vi "Output Wrist.vi"(11 "TeleOp Data Cluster":T1={"Drive Forward Input "=0.0, "Drive Twist Input"=0.0, "Drive Output"=0.0, "Drivetwist Output"=0.0, "Left Joystick Buttons"=[], "Left Joystick Axis"=[], "Right Joystick Axis"=[0.0, -0.007874015748031496, 0.0, -1.0], "Right Joystick Button"=[FALSE, FALSE, FALSE, FALSE, FALSE, FALSE, FALSE, FALSE, FALSE, FALSE, FALSE, FALSE], "Arm Encoder"=-20.0, "Left Drive Encoder"=0.0, "Right Drive Encoder"=36963.0, "Gyro Angle "=16.259765625, "Arm Joystick Output  "=-0.003937007874015748, "Line Follower L, C, R "=[TRUE, TRUE, TRUE], "Line follow?"=FALSE, " Climb Solenoid"=FALSE, "Wrist Encoder Count"=0.0, "Wrist Joystick Output"=0.0, "Ball Encoder Count"=0.0, "Ball Output"=0.0, "Climb Encoder"=0.0, "Climb Motor Output"=0.0, " Hatch Solenoid"=FALSE, "Arm Setpoint "=6.0, "Wrist Setpoint "=0.0, "Arm Joystick Enabled?"=FALSE, "Wrist Joystick Enabled"=FALSE, "Vision String"="0, 0, 0, 0, 0, 0", "Left Joystick POVs"=[]}) -> ()   [LabVIEW 2018]
uses:
  TypeDefs/Teleop Data Cluster.ctl
  TypeDefs/typedef_enum_Refnums.ctl
  TypeDefs/Joystick Buttons.ctl
  <vilib>/Rock Robotics/WPI/ThirdParty/Phoenix-LabVIEW/Motor Controller/Controls/CTRE_Phoenix_MotorControl_ControlMode.ctl
  <vilib>/Rock Robotics/WPI/ThirdParty/Phoenix-LabVIEW/Motor Controller/Get/CTRE_Phoenix_MotorController_GetLimitSwitchStates.vi
  <vilib>/Rock Robotics/Network Tables/NT Write Number.vi
  <vilib>/Rock Robotics/WPI/ThirdParty/Phoenix-LabVIEW/Motor Controller/Get/CTRE_Phoenix_MotorController_GetVoltage.vi
  <vilib>/Rock Robotics/WPI/ThirdParty/Phoenix-LabVIEW/Motor Controller/Get/CTRE_Phoenix_MotorController_GetClosedLoopData.vi
  <vilib>/Rock Robotics/WPI/ThirdParty/Phoenix-LabVIEW/Motor Controller/Get/CTRE_Phoenix_MotorController_GetSelectedSensorData.vi
  <vilib>/Rock Robotics/Network Tables/NT Write Boolean.vi
  <vilib>/ptbypt/NI_PtbyPt.lvlib
panel:
  in  "test setpt":i32
  in  "Setpoint 0":i32=-75
  in  "Top: Button; Bot: test":bool=TRUE
  in  "Setpoint 2":i32=600
  in  "Setpoint 1":i32=100
  out "Angle Out":dbl=22.5
  out "velocity Chart":i32(graph)
  out "Encoder Count":dbl
  out "Quadrature Velocity":i32
  in  "joystick scale factor":dbl=0.3
  in  "joystick upper limit":dbl=0.3 format="%#_13g"
  in  "joystick lower limit":dbl=-0.3 format="%#_13g"
  in  "P":dbl
  in  "I":dbl
  in  "D":dbl
  in  "slotIdx":i32
  out "Encoder Graph":dbl[][](graph)=[[-75.0, 0.0]]
  out "Closed-loop Error":i32=-75
  out "Error Derivative":dbl
  out "Integral Accumulator":dbl=-4611840.0
  out "Closed-loop Target":dbl=-0.075
  out "Percent Output":dbl
  in  "Cruise Angular Velocity raw":dbl=200.0 format="%#_13g"
  in  "Maximum Angular Accel raw":dbl=500.0 format="%#_13g"
  out "Closed Loop Target (deg)":dbl=-50.00164794921875
  out "Closed Loop Error (deg)":dbl=-51.64794921875
  in  "F":dbl
  in  "Arbitrary Feed Forward at 0":dbl
  in  "dt":u32
  in  "Reset Encoder":bool
  in  "joystick control? OR Thumb":bool
  # "top:  button mode"
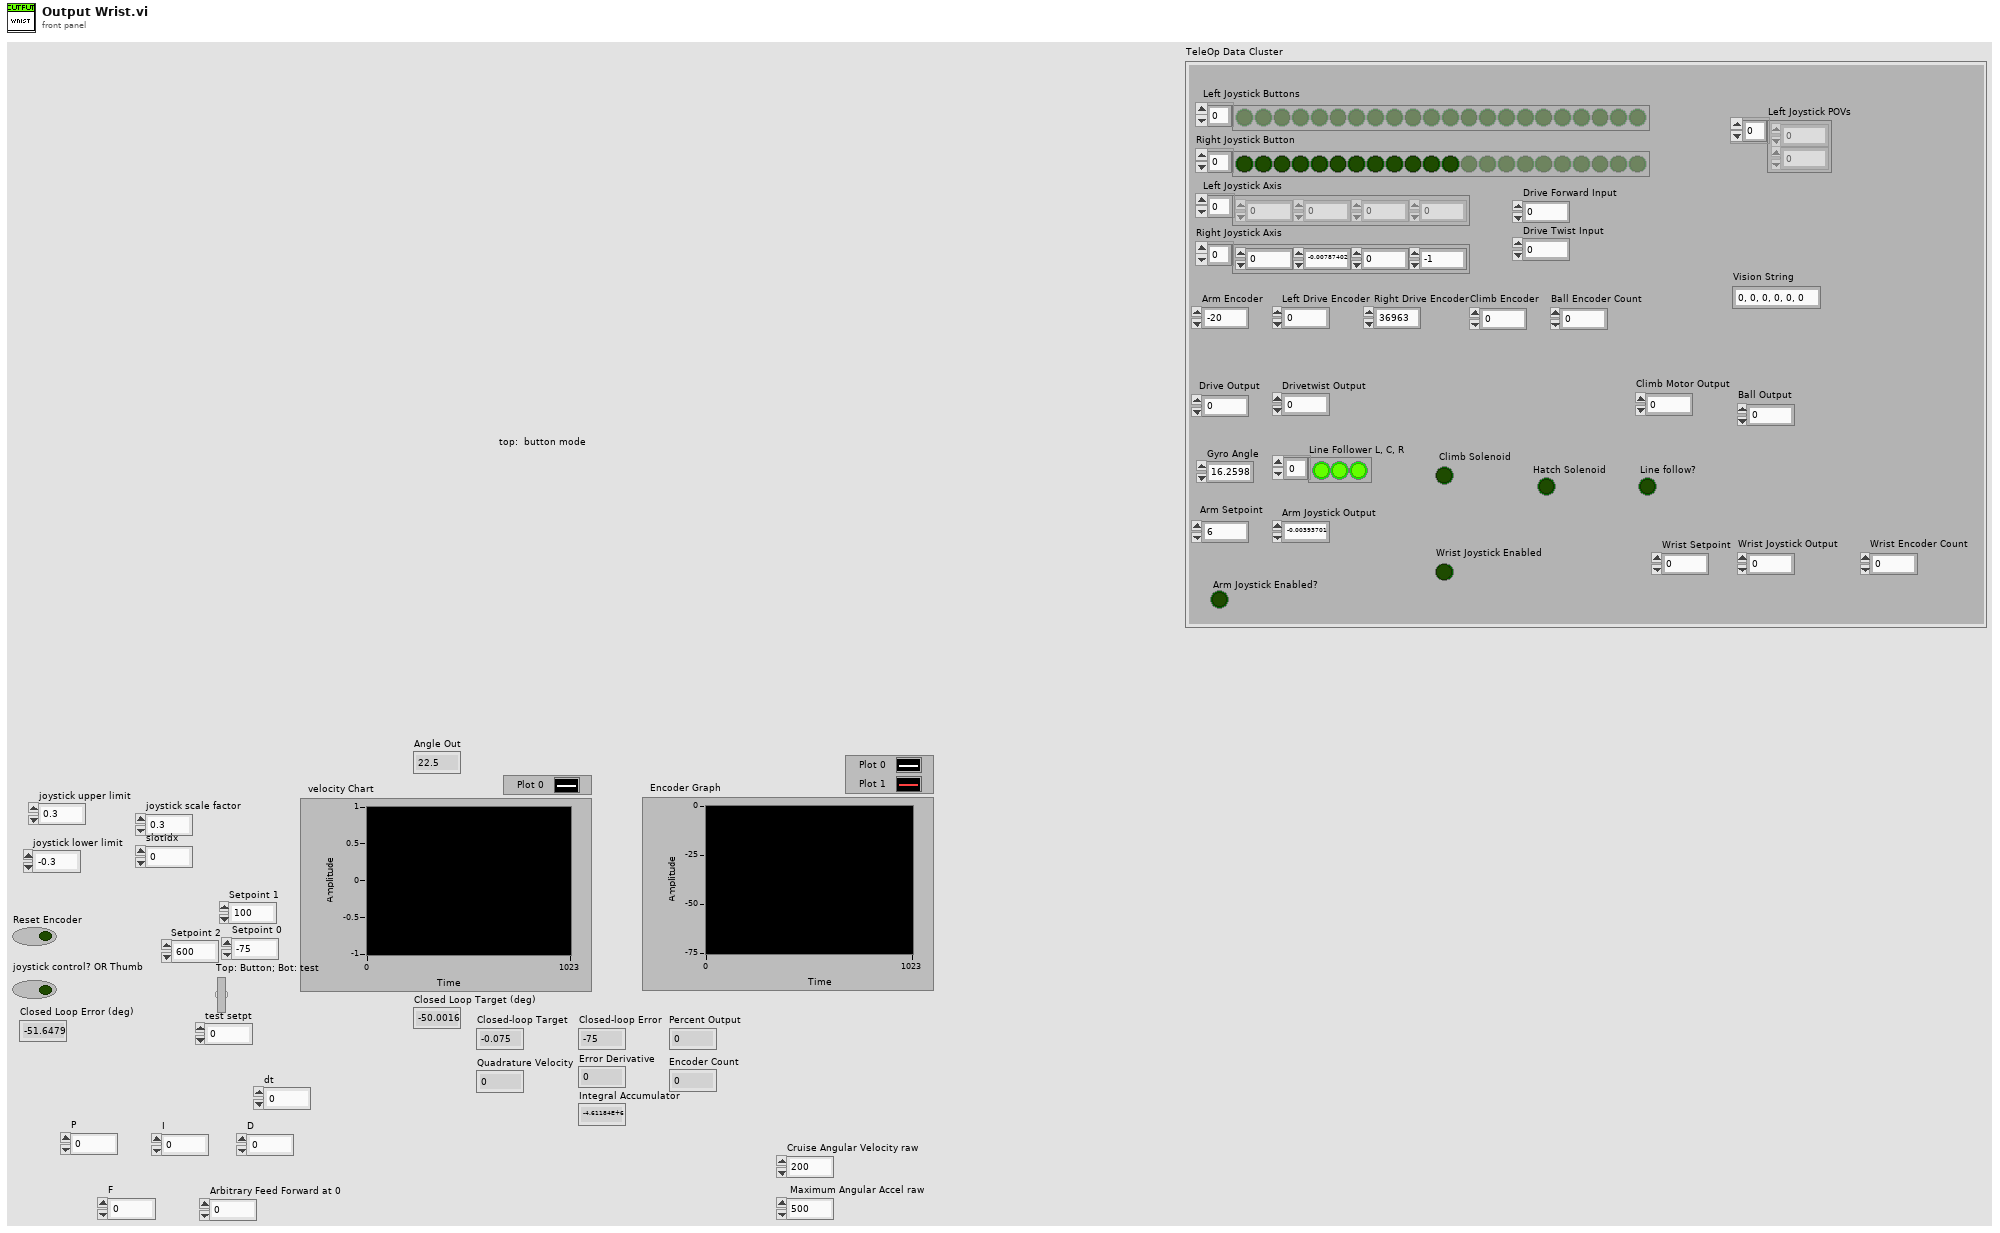
[diagram p1: front panel]
types:
  T1 = typedef "Teleop Data Cluster.ctl" = cluster{"Drive Forward Input ":dbl, "Drive Twist Input":dbl, "Drive Output":dbl, "Drivetwist Output":dbl, "Left Joystick Buttons":bool[], "Left Joystick Axis":dbl[], "Right Joystick Axis":dbl[], "Right Joystick Button":bool[], "Arm Encoder":dbl, "Left Drive Encoder":dbl, "Right Drive Encoder":dbl, "Gyro Angle ":dbl, "Arm Joystick Output  ":dbl, "Line Follower L, C, R ":bool[], "Line follow?":bool, " Climb Solenoid":bool, "Wrist Encoder Count":dbl, "Wrist Joystick Output":dbl, "Ball Encoder Count":dbl, "Ball Output":dbl, "Climb Encoder":dbl, "Climb Motor Output":dbl, " Hatch Solenoid":bool, "Arm Setpoint ":dbl, "Wrist Setpoint ":dbl, "Arm Joystick Enabled?":bool, "Wrist Joystick Enabled":bool, "Vision String":string, "Left Joystick POVs":i16[]}
  T2 = typedef "Joystick Buttons.ctl" = enum16{"Trigger", "Thumb", "Top 3", "Top 4", "Top 5", "Top 6", "Bottom 7", "Bottom 8", "Bottom 9", "Bottom 10", "Bottom 11", "Bottom 12"}
  T3 = typedef "typedef_enum_Refnums.ctl" = enum16{"Ball_Encoder", "Ball_Motor", "Camera", "Linefollow_3", "Linefollow_2", "Linefollow_1", "Gyro", "Hatch_Solenoid", "Climb_Back_Solenoid", "Arm_Encoder", "Arm_Motor", "Lift_Encoder", "Drive", "Drive_Motor_R", "Drive_Motor_L", "Drive_Encoder_R", "Drive_Encoder_L", "Joy_R", "Joy_L", "Wrist_Motor", "Wrist_Encoder", "Climb Upper Limit", "Climb Lower Limit ", "Climb_Front_Motor"}
  T4 = typedef "WPI_MotorControlDeviceRef.ctl" = cluster{"DeviceStatus":errorcluster, "Type":T5, "PWM":cluster{"PWM Channel":T6, "DeadBand":T7}, "CAN":cluster{"Device Number":u8, "SetOutput VI Ref":variant, "GetOutput VI Ref":variant, "Enable VI Ref":variant, "Disable VI Ref":variant, "Data":variant}, "Invert":bool, "DIO PWM":cluster{"PWM \"Enable\" Channel":T6, "DIOChannel":T8, "PWM Rate":dbl}}
  T5 = typedef "WPI_MotorControlType.ctl" = enum16{"PWM", "CAN", "DIO PWM"}
  T6 = typedef "FPGA_DIOPWMChannel.ctl" = enum8{"PWM 0", "PWM 1", "PWM 2", "PWM 3", "PWM 4", "PWM 5", "PWM 6", "PWM 7", "PWM 8", "PWM 9", "PWM MXP 0", "PWM MXP 1", "PWM MXP 2", "PWM MXP 3", "PWM MXP 4", "PWM MXP 5", "PWM MXP 6", "PWM MXP 7", "PWM MXP 8", "PWM MXP 9", "Invalid"}
  T7 = typedef "WPI_PWMDeadband.ctl" = cluster{"Name":string, "maxPositivePwm":i32, "minPositivePwm":i32, "centerPwm":i32, "maxNegativePwm":i32, "minNegativePwm":i32, "angularRange":u16}
  T8 = typedef "FPGA_DIOChannel.ctl" = enum8{"DIO 0", "DIO 1", "DIO 2", "DIO 3", "DIO 4", "DIO 5", "DIO 6", "DIO 7", "DIO 8", "DIO 9", "DIO MXP 0", "DIO MXP 1", "DIO MXP 2", "DIO MXP 3", "DIO MXP 4", "DIO MXP 5", "DIO MXP 6", "DIO MXP 7", "DIO MXP 8", "DIO MXP 9", "DIO MXP 10", "DIO MXP 11", "DIO MXP 12", "DIO MXP 13", "DIO MXP 14", "DIO MXP 15", "SPI Port CS1", "SPI Port CS2", "SPI Port CS3", "SPI Port MISO", "SPI Port MOSI", "Invalid"}
  T9 = enum16{"DemandType_Neutral", "DemandType_AuxPID", "DemandType_ArbitraryFeedForward"}
  T10 = typedef "CTRE_Phoenix_MotorControl_ControlMode.ctl" = u16
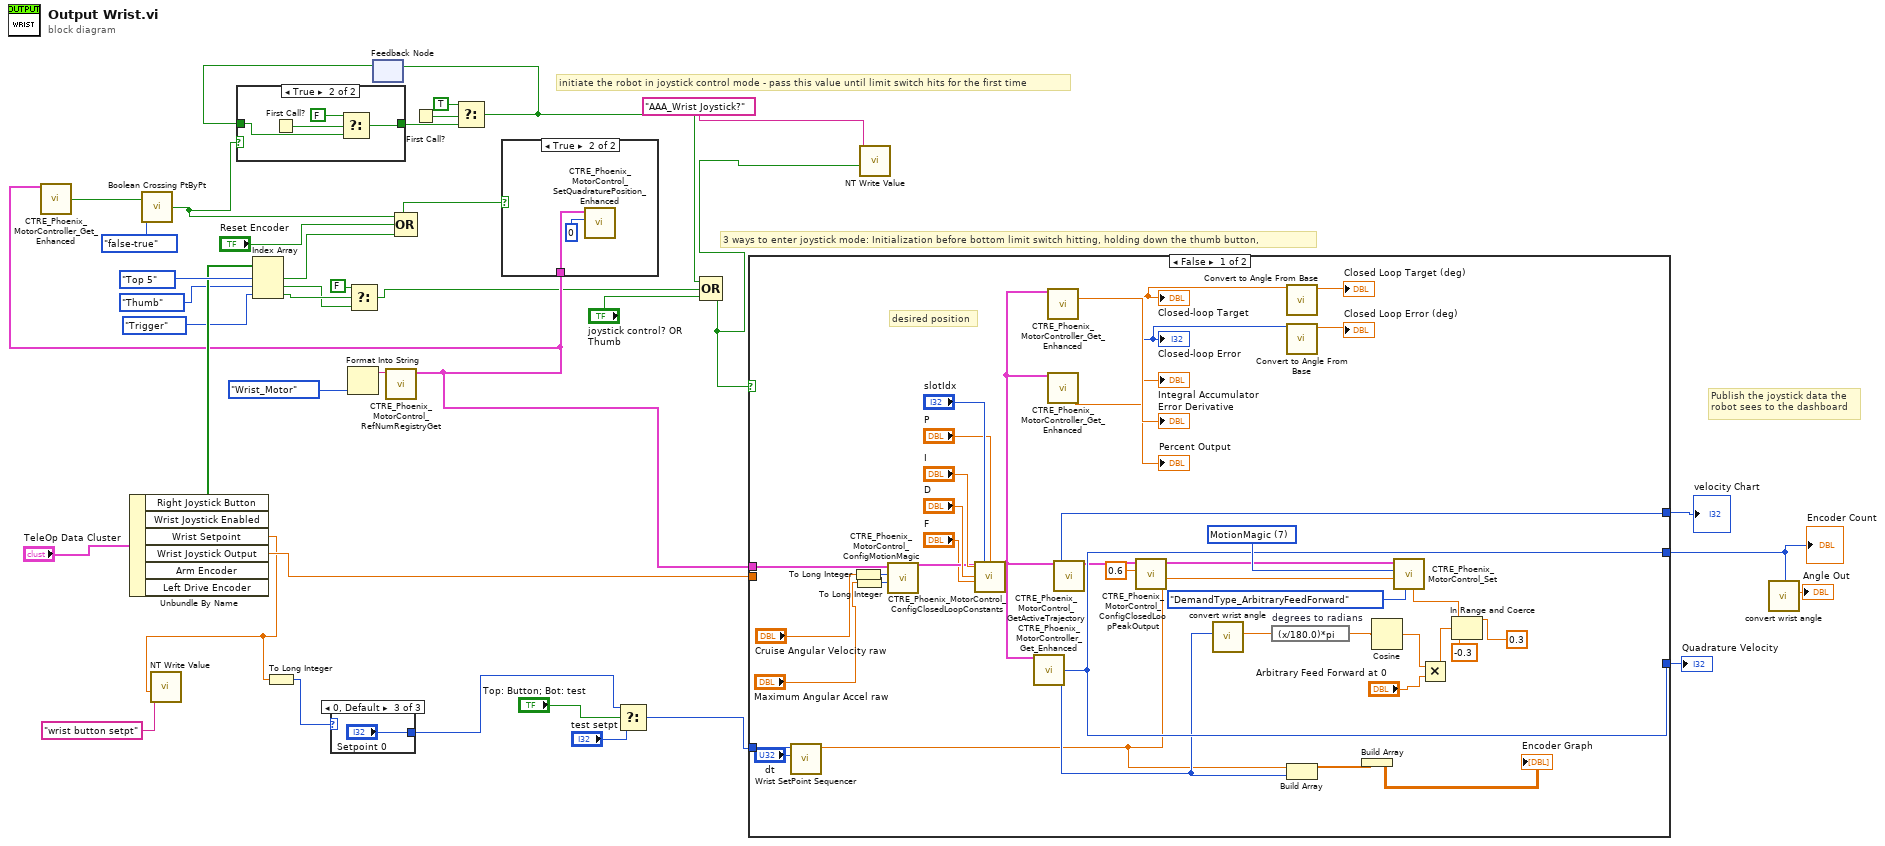
[diagram p0: block diagram]
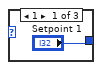
[diagram p3: hidden frame]
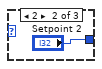
[diagram p4: hidden frame]
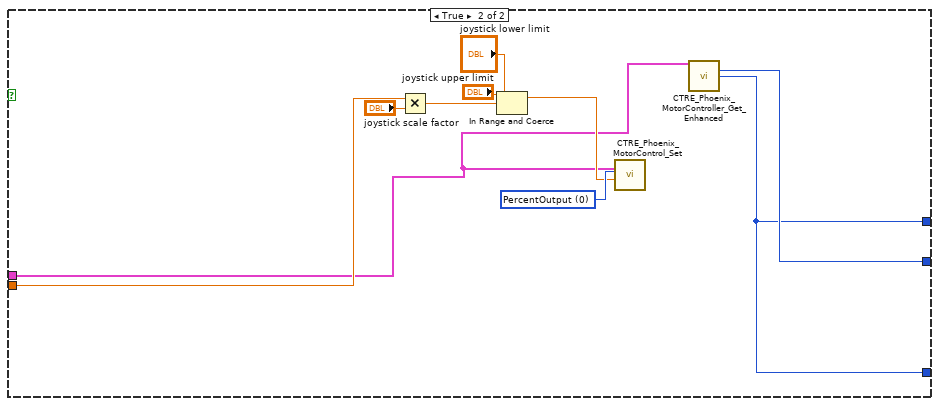
[diagram p5: hidden frame]
diagram:
  # "3 ways to enter joystick mode: Initialization before bottom limit switch hitting, holding down the thumb button,"
  # "initiate the robot in joystick control mode - pass this value until limit switch hits for the first time"
  # "Publish the joystick data the\nrobot sees to the dashboard"
  n1 = Unbundle By Name("TeleOp Data Cluster") -> ("Right Joystick Button"=w34:bool[], "Wrist Setpoint"=w24:dbl, "Wrist Joystick Output"=w28:dbl)  [unwired: 3 out]
  n2 = call-poly <vilib>:"NT Write Value.vi"("Numeric"=w24, "Name"="wrist button setpt") -> ()  [unwired: 9 in, 1 out]
  n3 = Index Array(array=w34, index #1=Joystick_Buttons."Top 5" ("Enum"), index #2=Joystick_Buttons."Thumb" ("Enum"), index #3=Joystick_Buttons."Trigger" ("Enum")) -> (element #1=w19:bool, element #2=w6:bool, element #3=w7:bool)
  n4 = To Long Integer(number=w24) -> (32bit integer=w23:i32)
  n5 = case shown="0, Default" w23 {
    tunnel: ["Setpoint 1" "Setpoint 2" "Setpoint 0"] -> w26
    frame 1 {
    }
    frame 2 {
    }
    frame 0, Default {
    }
  }
  n6 = Format Into String(typedef_enum_Refnums."Wrist_Motor" ("RefNums")) -> (resulting string=w37:string)  [unwired: 3 in, 1 out]
  n7 = Select(t=FALSE, s=w7, f=w6) -> (s? t:f=w4:bool)
  n8 = feedback #1() -> (w15:bool)  [unwired: 1 in]
  n9 = call <vilib>:"CTRE_Phoenix_MotorControl_RefNumRegistryGet.vi"("refnum name"=w37) -> ("PhoenixMotorControlDevRef"=w20:T4)  [unwired: 9 in, 1 out]
  n10 = call-poly <vilib>:"CTRE_Phoenix_MotorController_Get_Enhanced.vi"("PhoenixMotorControlDevRef"=w20) -> ("Reverse Limit Closed?"=w1:bool)  [unwired: 11 in, 3 out]
  n11 = call <vilib>:"Boolean Crossing PtByPt.vi"("direction"=enum16{"either", "false-true", "true-false"}."false-true", "input"=w1) -> ("crossing"=w17:bool)  [unwired: 1 in]
  n12 = case shown="True" w17 {
    tunnel: [w42 w43] -> w12
    tunnel: w15 -> [w42 w45]
    frame False {
    }
    frame True {
      n13 = First Call?() -> (First Call?: T/F=w46:bool)
      n14 = Select(t=FALSE, s=w46, f=w45) -> (s? t:f=w43:bool)
    }
  }
  n15 = Compound Arithmetic op=OR(w17, "Reset Encoder", w19) -> (w16:bool)
  n16 = First Call?() -> (First Call?: T/F=w14:bool)
  n17 = Select(t=TRUE, s=w14, f=w12) -> (s? t:f=w9:bool)
  n18 = feedback-in #1(w9) -> ()
  n19 = case shown="True" w16 {
    tunnel: w20 -> [_ w47]
    frame False {
    }
    frame True {
      n20 = call <vilib>:"CTRE_Phoenix_MotorControl_SetQuadraturePosition_Enhanced.vi"("New Position"=0, "PhoenixMotorControlDevRef"=w47) -> ()  [unwired: 8 in, 2 out]
    }
  }
  n21 = Select(t=w26, s="Top: Button; Bot: test", f="test setpt") -> (s? t:f=w22:i32)
  n22 = Compound Arithmetic op=OR(w9, w4, "joystick control? OR Thumb") -> (w3:bool)
  n23 = case shown="False" w3 {
    tunnel: [w76 w91] -> w32
    tunnel: [w78 w91] -> w31
    tunnel: [w76 w92] -> w30
    tunnel: w22 -> [w55 _]
    tunnel: w20 -> [w52 w89]
    tunnel: w28 -> [_ w90]
    frame False {
      w83 = T10 7 items=["PercentOutput"=0, "Position"=1, "Velocity"=2, "Current"=3, "Follower"=5, "MotionProfile"=6, "MotionMagic"=7, "MotionProfileArc"=10, "Disabled"=15] ("Control Mode")
      # "desired position"
      n24 = call "Wrist SetPoint Sequencer.vi"("dt"="dt", "SetPoint"=w55) -> ("Active SetPoint"=w54:dbl)  [unwired: 9 in]
      n25 = To Long Integer(number="Cruise Angular Velocity raw") -> (32bit integer=w74:i32)
      n26 = To Long Integer(number="Maximum Angular Accel raw") -> (32bit integer=w73:i32)
      n27 = call <vilib>:"CTRE_Phoenix_MotorControl_ConfigMotionMagic.vi"("Acceleration"=w73, "Cruise Velocity"=w74, "PhoenixMotorControlDevRef"=w52) -> ("PhoenixMotorControlDevRef"=w84:T4)  [unwired: 7 in, 1 out]
      n28 = call <vilib>:"CTRE_Phoenix_MotorControl_ConfigClosedLoopConstants.vi"("PhoenixMotorControlDevRef"=w84, "slotIdx"="slotIdx", "P"="P", "I"="I", "D"="D", "F"="F") -> ("PhoenixMotorControlDevRef"=w77:T4)  [unwired: 8 in, 1 out]
      n29 = call-poly <vilib>:"CTRE_Phoenix_MotorController_Get_Enhanced.vi"("PhoenixMotorControlDevRef"=w77) -> ("Position (Raw Sensor Units)"=w56:i32, "Velocity (Raw Sensor Units per 100 ms)"=w76:i32)  [unwired: 11 in, 2 out]
      n30 = call-poly <vilib>:"CTRE_Phoenix_MotorController_Get_Enhanced.vi"("PhoenixMotorControlDevRef"=w77) -> ("Closed-loop Target"=w71:dbl, "Closed-loop Error"=w68:i32, "Error Derivative"=→"Error Derivative":dbl, "Integral Accumulator"=→"Integral Accumulator":dbl)  [unwired: 9 in, 2 out]
      "Closed-loop Error" <- w68
      "Closed-loop Target" <- w71
      n31 = call-poly <vilib>:"CTRE_Phoenix_MotorController_Get_Enhanced.vi"("PhoenixMotorControlDevRef"=w77) -> ("Percent Output"=→"Percent Output":dbl)  [unwired: 10 in, 4 out]
      n32 = call <vilib>:"CTRE_Phoenix_MotorControl_GetActiveTrajectory.vi"("PhoenixMotorControlDevRef"=w77) -> ("PhoenixMotorControlDevRef"=w51:T4, "Velocity (Sensor Units per 100 ms)"=w78:i32)  [unwired: 10 in, 3 out]
      n33 = call <vilib>:"CTRE_Phoenix_MotorControl_ConfigClosedLoopPeakOutput.vi"("peakOutput"=0.6, "PhoenixMotorControlDevRef"=w51) -> ("PhoenixMotorControlDevRef"=w50:T4)  [unwired: 8 in, 1 out]
      n34 = call "convert wrist angle.vi"("Horizontal Encoder Ct"=w56) -> ("Angle Out"=w58:dbl)  [unwired: 9 in, 1 out]
      n35 = expression code="(x/180.0)*pi" "degrees to radians"(w58) -> (w62:dbl)
      n36 = call "Convert to Angle From Base.vi"("Horizontal Encoder Ct"=w71) -> ("Angle Out"=→"Closed Loop Target (deg)":dbl)  [unwired: 9 in, 1 out]
      n37 = call "Convert to Angle From Base.vi"("Horizontal Encoder Ct"=w68) -> ("Angle Out"=→"Closed Loop Error (deg)":dbl)  [unwired: 9 in, 1 out]
      n38 = Build Array(w54, w56) -> (w72:dbl[])
      n39 = Build Array(w72) -> (→"Encoder Graph":dbl[][])
      n40 = Cosine(x=w62) -> (cos(x)=w61:dbl)
      n41 = Multiply(x=w61, y="Arbitrary Feed Forward at 0") -> (x*y=w57:dbl)
      n42 = In Range and Coerce(upper limit=0.3, x=w57, lower limit=-0.3) -> (coerced(x)=w63:dbl)  [unwired: 1 out]
      n43 = call <vilib>:"CTRE_Phoenix_MotorControl_Set.vi"("Demand1"=w63, "DemandType"=T9."DemandType_ArbitraryFeedForward", "Output"=w54, "Control Mode"=w83, "PhoenixMotorControlDevRef"=w50) -> ()  [unwired: 5 in, 2 out]
    }
    frame True {
      w98 = T10 0 items=["PercentOutput"=0, "Position"=1, "Velocity"=2, "Current"=3, "Follower"=5, "MotionProfile"=6, "MotionMagic"=7, "MotionProfileArc"=10, "Disabled"=15] ("Control Mode")
      n44 = Multiply(x=w90, y="joystick scale factor") -> (x*y=w95:dbl)
      n45 = In Range and Coerce(upper limit="joystick upper limit", x=w95, lower limit="joystick lower limit") -> (coerced(x)=w94:dbl)  [unwired: 1 out]
      n46 = call <vilib>:"CTRE_Phoenix_MotorControl_Set.vi"("Output"=w94, "Control Mode"=w98, "PhoenixMotorControlDevRef"=w89) -> ()  [unwired: 7 in, 2 out]
      n47 = call-poly <vilib>:"CTRE_Phoenix_MotorController_Get_Enhanced.vi"("PhoenixMotorControlDevRef"=w89) -> ("Position (Raw Sensor Units)"=w92:i32, "Velocity (Raw Sensor Units per 100 ms)"=w91:i32)  [unwired: 11 in, 2 out]
    }
  }
  "Quadrature Velocity" <- w32
  "Encoder Count" <- w30
  "velocity Chart" <- w31
  n48 = call-poly <vilib>:"NT Write Value.vi"("Boolean"=w3, "Name"="AAA_Wrist Joystick?") -> ()  [unwired: 9 in, 1 out]
  n49 = call "convert wrist angle.vi"("Horizontal Encoder Ct"=w30) -> ("Angle Out"=→"Angle Out":dbl)  [unwired: 9 in, 1 out]
